vi "TimeResolvedSpectroscopy.vi"() -> ()   [LabVIEW 2016]
uses:
  C:/Users/VaidaLabAdmin/Desktop/CodyEthanJordan/LaserControl/DelayStageDlls/Thorlabs.MotionControl.Controls.dll
  DelayStageDlls/Thorlabs.MotionControl.Controls.dll
  C:/Users/VaidaLabAdmin/Desktop/CodyEthanJordan/LaserControl/DelayStageDlls/Thorlabs.MotionControl.Benchtop.BrushlessMotorCLI.dll
  DelayStageDlls/Thorlabs.MotionControl.Benchtop.BrushlessMotorCLI.dll
  C:/Users/VaidaLabAdmin/Desktop/CodyEthanJordan/LaserControl/DelayStageDlls/Thorlabs.MotionControl.GenericMotorCLI.dll
  DelayStageDlls/Thorlabs.MotionControl.GenericMotorCLI.dll
panel:
  out "Start Time":string="120419_1643"
  out "RoiSum":dbl=1907.0
  in  "Main UI":T1(tab)=enum."Collect Data"
  in  "BenchtopBrushlessControl 3":refnum<k24>(container)
  in  "SerialNumber":string="73871558"
  out "Settings":T2={"Range"=5056, "cftfak"=39321856, "RoiMin"=0, "RoiMax"=4096, "#Regions"=0, "Caluse"=1, "Calpoints"=0, "Param"=0, "Offset"=0, "Xdim"=0, "bitshift"=0, "Active"=1, "Roipreset"=0.0, "dummy1"=0.0, "dummy2"=0.0, "dummy3"=0.0} {"dummy3" format="%.2f"; "dummy2" format="%.2f"; "bitshift" format="%.0x"; "Active" format="%.0x"; "Offset" format="%.0x"; "Param" format="%.0x"; "dummy1" format="%.2f"; "Roipreset" format="%.2f"; "cftfak" format="%.0x"}
  in  "Maximum Scan\nPosition":dbl=3000.0
  out "Harmonics":cluster{"Y":dbl[], "Y":dbl[]}[](graph)=[{"Y"=[20.0], "Y"=[1907.0]}]
  in  "Start Scan":bool
  out "Spectrum":u32[](graph)
  in  "State":T3(ring)=enum."Move Grating"
  out "Delay Position":dbl=20.0
  in  "Step Size":dbl=10.0
  in  "Sweeps":i32=3000
  out "CHN Status":T4={"Started"=3, "Maxval"=0, "Runtime"=0.101, "Fifo full"=0.0, "TotalSum"=2383.0, "RoiSum"=1907.0, "Roirate"=5639.14373088685, "Sweeps"=3005.0, "Starts"=0.0, "Dummy"=0.0} {"Dummy" format="%.2f"; "Starts" format="%.2f"; "Sweeps" format="%.2f"; "Roirate" format="%.2f"; "RoiSum" format="%.2f"; "TotalSum" format="%.2f"; "Fifo full" format="%.2f"; "Runtime" format="%.2f"}
  in  "Photoelectron Spectra Destination":path=path "C:/Users/VaidaLabAdmin/Documents/TOF-PES/04-12-2019/test"
  out "Halt Confirmation":string="OK"
  out "MCSADat Error":i32
  in  "Spectrum #":i32
  in  "Stop":bool
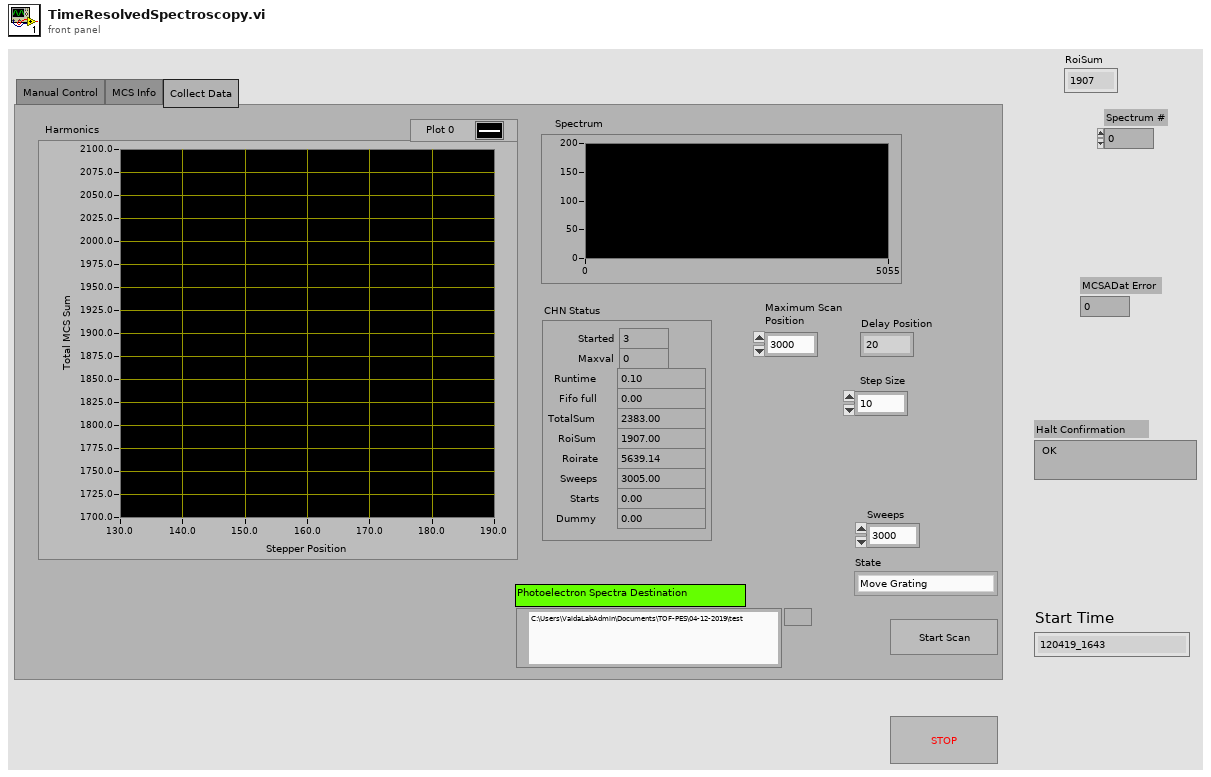
[diagram p1: front panel]
types:
  T1 = enum32{"Manual Control", "MCS Info", "Collect Data"}
  T2 = cluster{"Range":i32, "cftfak":i32, "RoiMin":i32, "RoiMax":i32, "#Regions":i32, "Caluse":i32, "Calpoints":i32, "Param":i32, "Offset":i32, "Xdim":i32, "bitshift":i32, "Active":i32, "Roipreset":dbl, "dummy1":dbl, "dummy2":dbl, "dummy3":dbl}
  T3 = enum16{"Start", "Move Grating", "Start MCS", "Collect Data", "Stop MCS", "Save Data", "Stop"}
  T4 = cluster{"Started":i32, "Maxval":u32, "Runtime":dbl, "Fifo full":dbl, "TotalSum":dbl, "RoiSum":dbl, "Roirate":dbl, "Sweeps":dbl, "Starts":dbl, "Dummy":dbl}
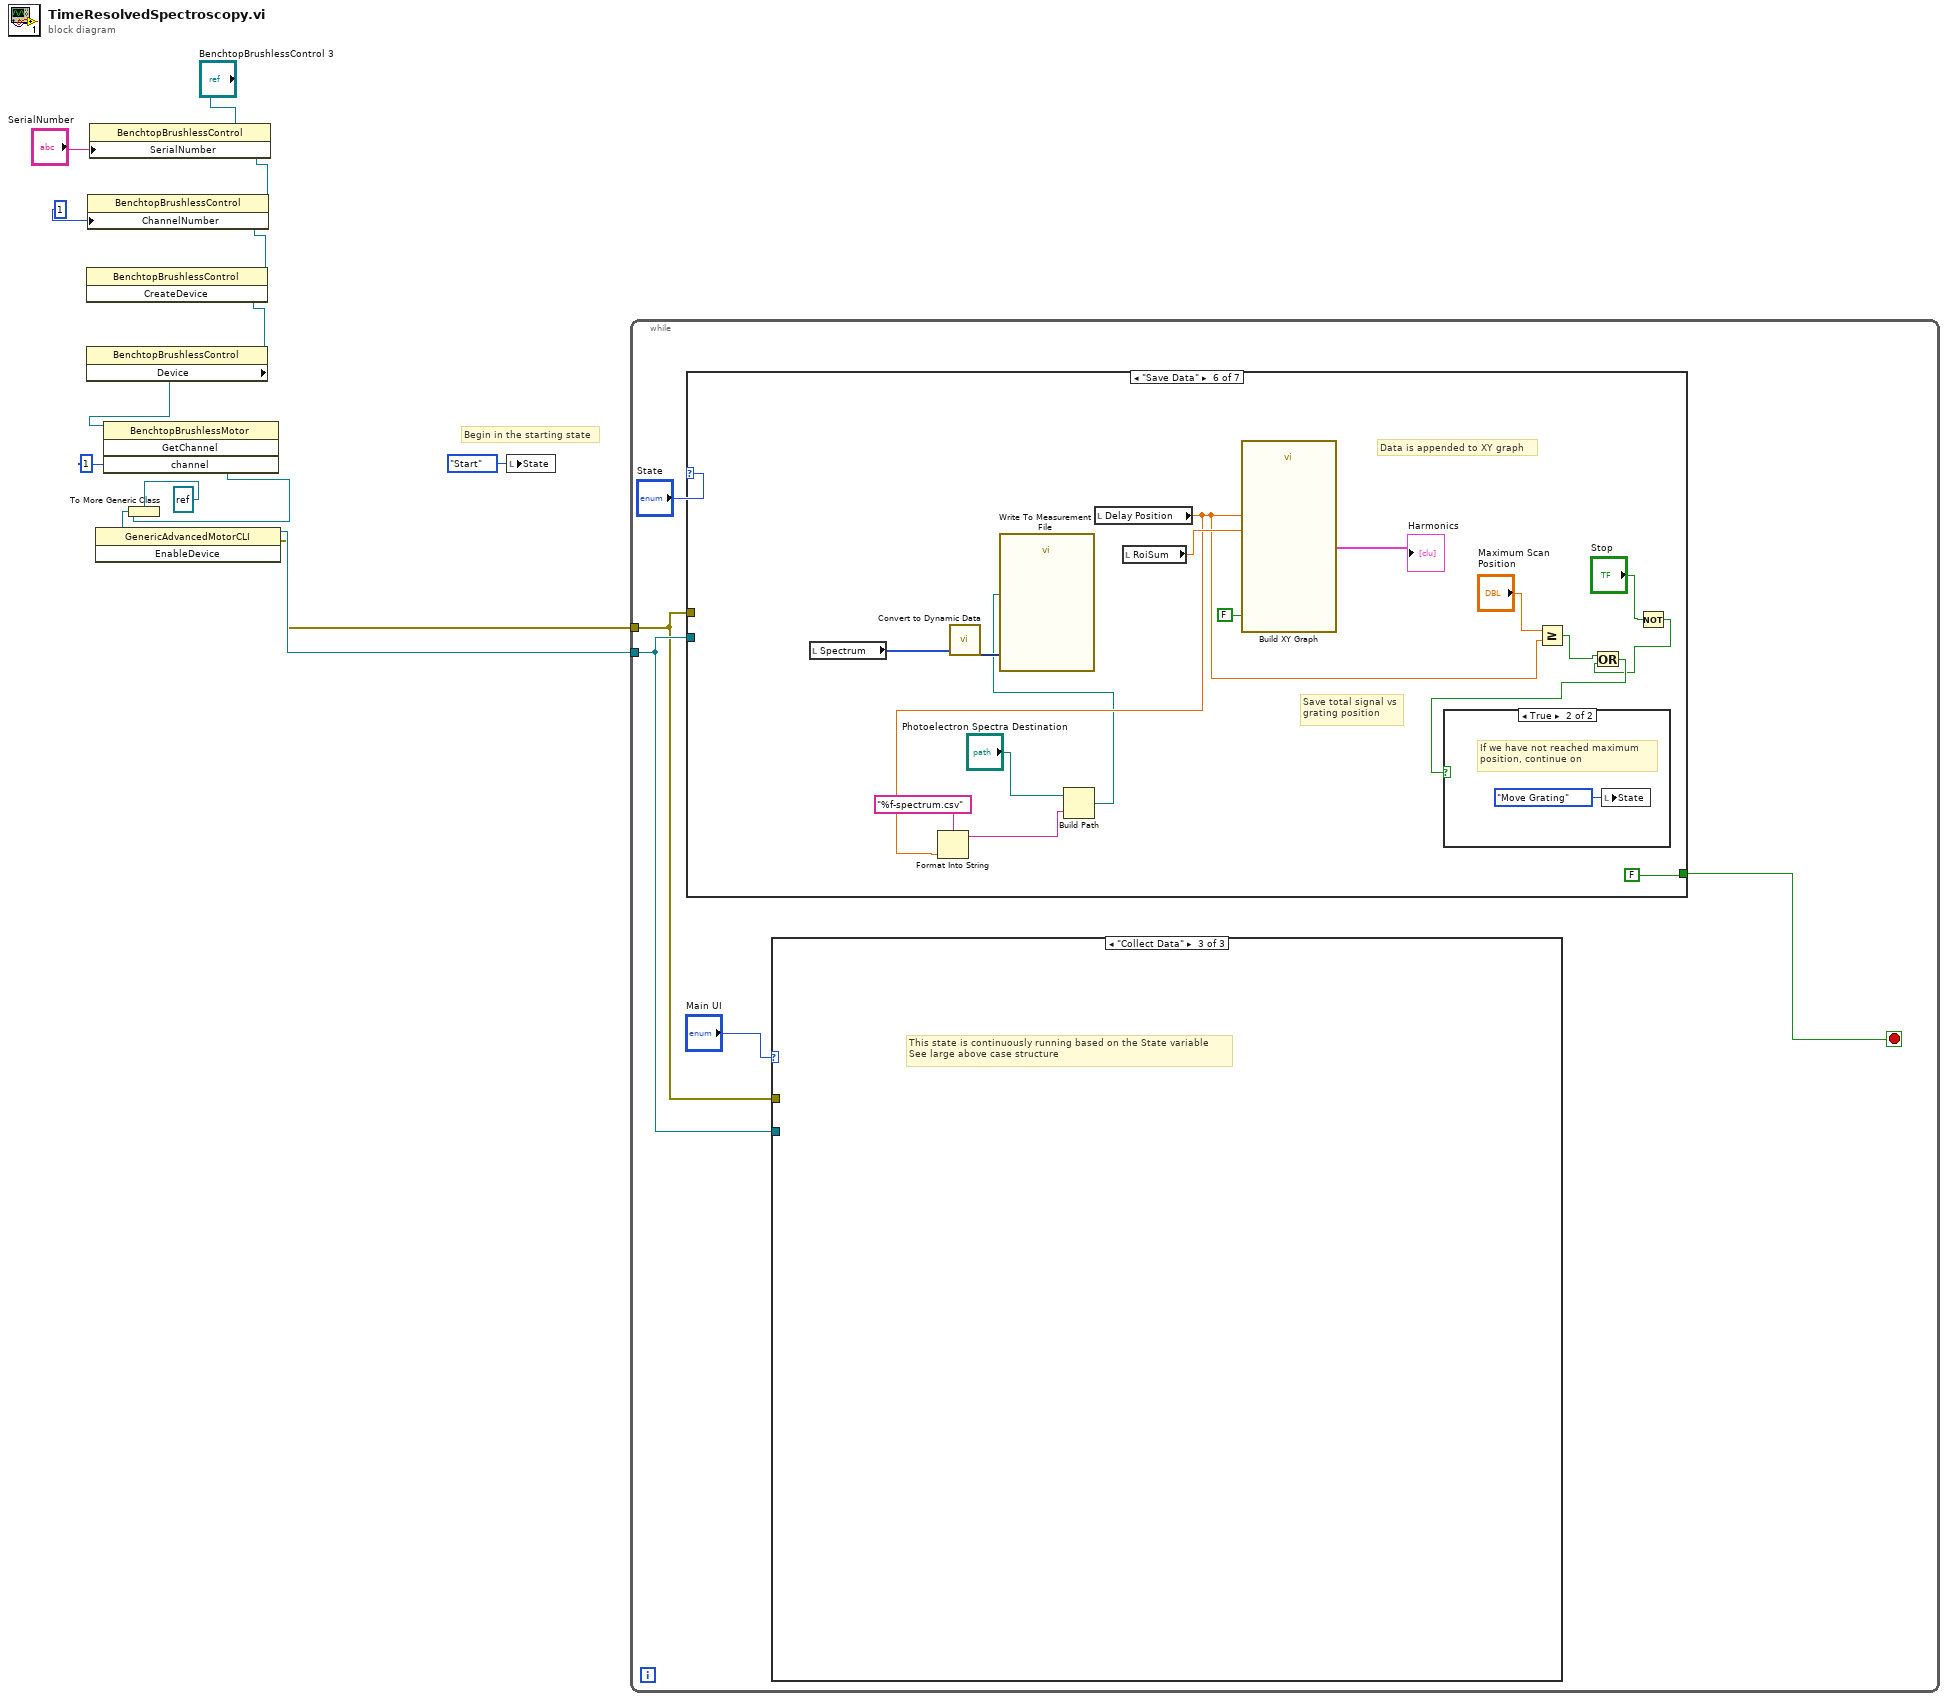
[diagram p0: block diagram]
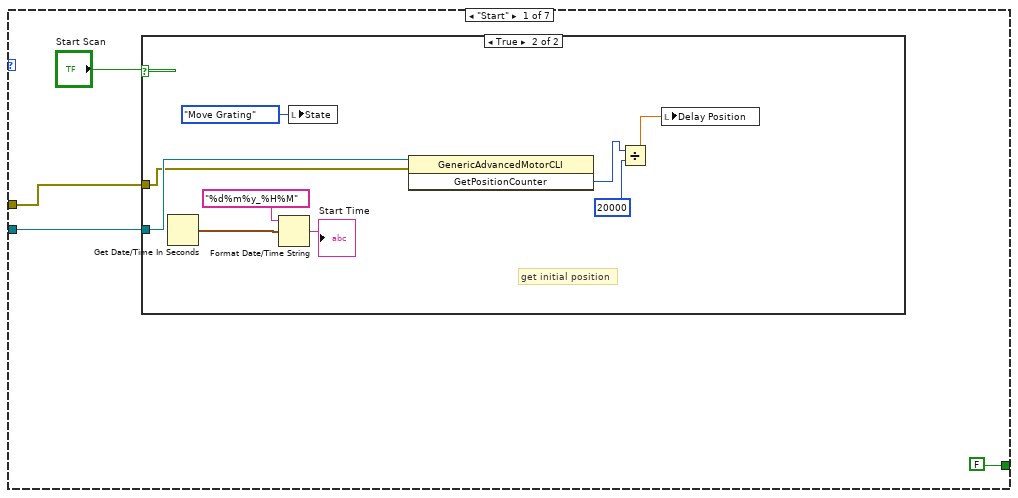
[diagram p4: hidden frame]
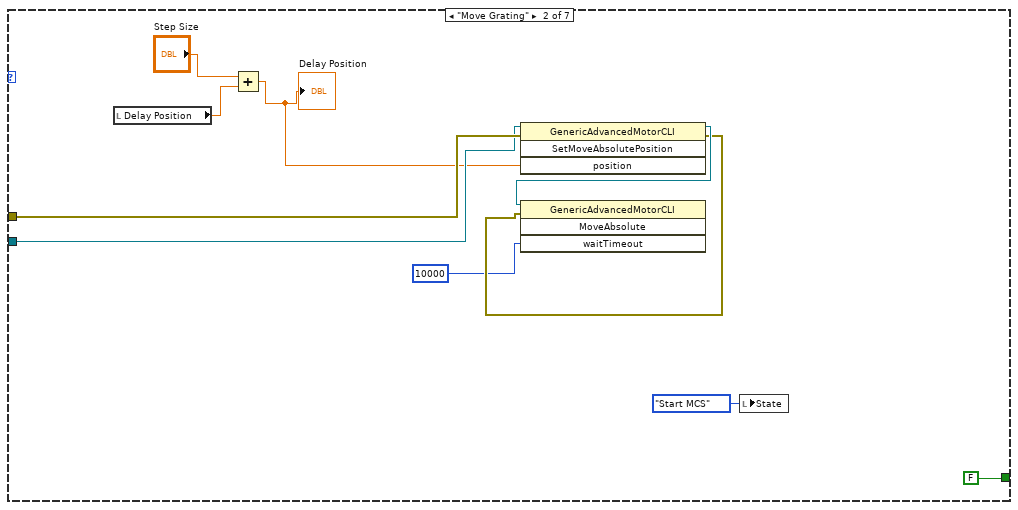
[diagram p6: hidden frame]
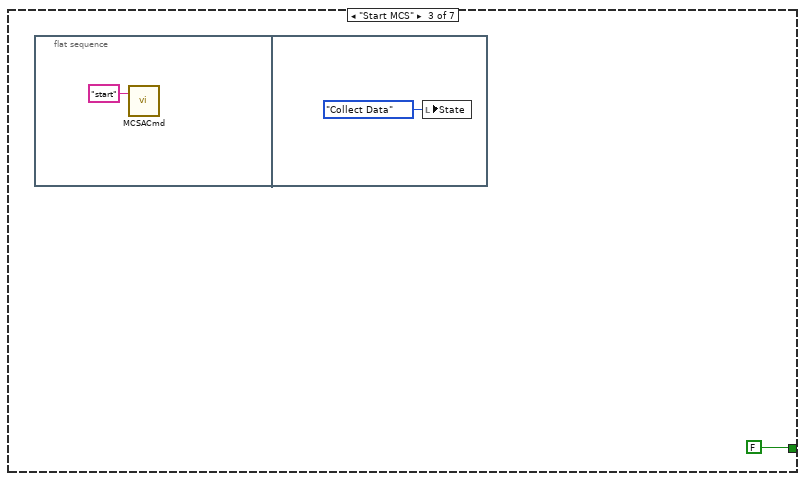
[diagram p7: hidden frame]
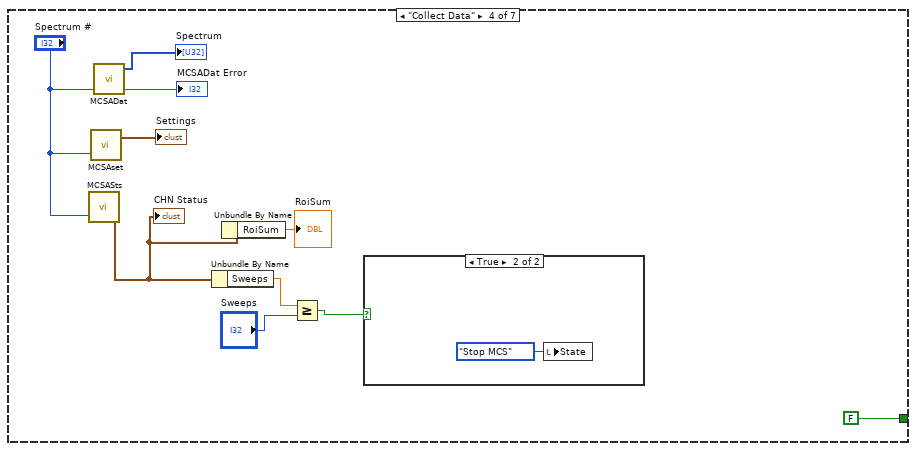
[diagram p8: hidden frame]
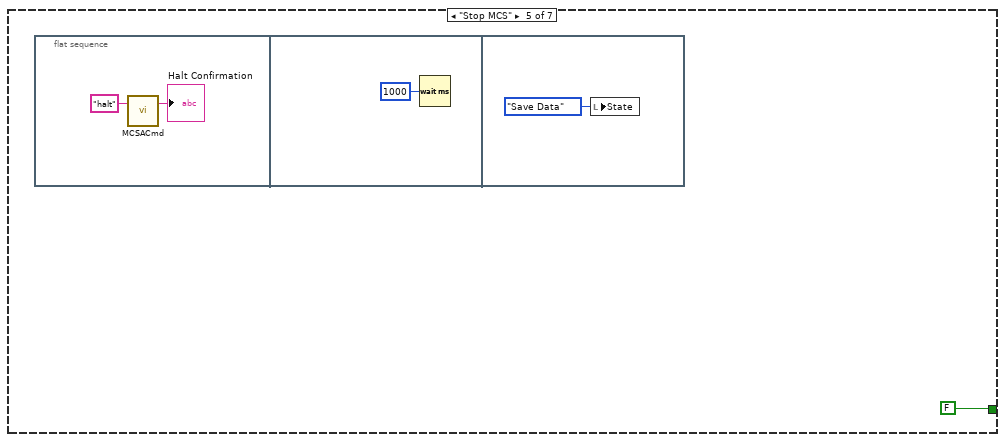
[diagram p10: hidden frame]
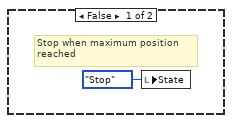
[diagram p11: hidden frame]
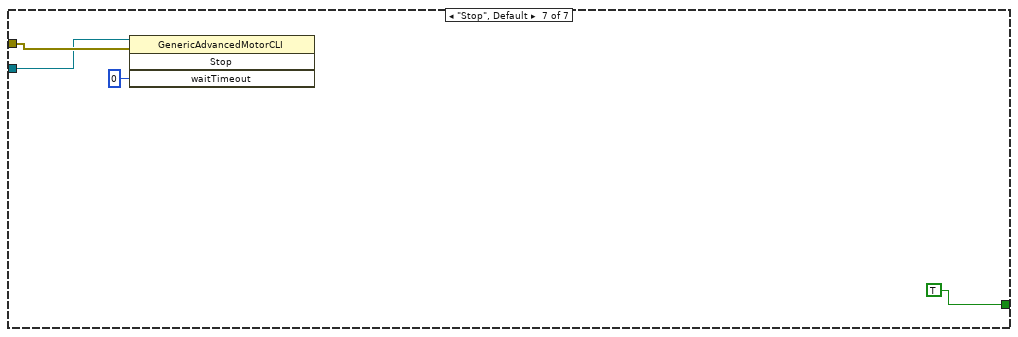
[diagram p12: hidden frame]
diagram:
  # "Begin in the starting state"
  n1 = property class="BenchtopBrushlessControl"(reference="BenchtopBrushlessControl 3", "SerialNumber"="SerialNumber") -> (reference out=w9:refnum<k24>)  [unwired: 1 in, 1 out]
  n2 = property class="BenchtopBrushlessControl"(reference=w9, "ChannelNumber"=1) -> (reference out=w8:refnum<k24>)  [unwired: 1 in, 1 out]
  n3 = invoke class="BenchtopBrushlessControl" method="CreateDevice"(reference=w8) -> (reference out=w7:refnum<k24>)  [unwired: 2 in, 2 out]
  n4 = property class="BenchtopBrushlessControl"(reference=w7) -> ("Device"=w6:refnum<k24>)  [unwired: 1 in, 2 out]
  n5 = invoke class="BenchtopBrushlessMotor" method="GetChannel"(reference=w6, "channel"=i16 1) -> ("GetChannel"=w4:refnum<k24>)  [unwired: 2 in, 3 out]
  n6 = To More Generic Class(target class=refnum<k24> refnum, reference=w4) -> (generic class reference=w5:refnum<k24>)
  n7 = invoke class="GenericAdvancedMotorCLI" method="EnableDevice"(reference=w5) -> (reference out=w2:refnum<k24>, error out=w1:errorcluster)  [unwired: 2 in, 1 out]
  n8 = local write "State"(T3."Start" ("State")) -> ()
  n9 = while {
    tunnel: w1 -> [w16]
    tunnel: w2 -> [w17]
    stop <- w15 stop-if-true
    n10 = case shown="\"Save Data\"" "State" {
      tunnel: w16 -> [w21 w38 _ _ _ _ w82]
      tunnel: w17 -> [w20 w36 _ _ _ _ w81]
      tunnel: [FALSE FALSE FALSE FALSE FALSE FALSE TRUE] -> w15
      frame "Start" {
        n11 = case shown="True" "Start Scan" {
          tunnel: w21 -> [_ w27]
          tunnel: w20 -> [_ w28]
          frame False {
          }
          frame True {
            # "get initial position"
            n12 = Get Date/Time In Seconds() -> (seconds since 1Jan1904=w30:timestamp)
            n13 = Format Date/Time String(time format string (%c)="%d%m%y_%H%M", seconds (now)=w30) -> (date/time string=→"Start Time":string)  [unwired: 1 in]
            n14 = local write "State"(T3."Move Grating" ("State")) -> ()
            n15 = invoke class="GenericAdvancedMotorCLI" method="GetPositionCounter"(reference=w28, error in=w27) -> ("GetPositionCounter"=w25:i32)  [unwired: 1 in, 2 out]
            n16 = Divide(x=w25, y=20000) -> (x/y=w26:dbl)
            n17 = local write "Delay Position"(w26) -> ()
          }
        }
      }
      frame "Move Grating" {
        n18 = local read "Delay Position"() -> (w41:dbl)
        n19 = Add(x="Step Size", y=w41) -> (x+y=w33:dbl)
        "Delay Position" <- w33
        n20 = invoke class="GenericAdvancedMotorCLI" method="SetMoveAbsolutePosition"(reference=w36, error in=w38, "position"=w33) -> (reference out=w39:refnum<k24>, error out=w37:errorcluster)  [unwired: 1 in, 2 out]
        n21 = invoke class="GenericAdvancedMotorCLI" method="MoveAbsolute"(reference=w39, error in=w37, "waitTimeout"=10000) -> ()  [unwired: 1 in, 4 out]
        n22 = local write "State"(T3."Start MCS" ("State")) -> ()
      }
      frame "Start MCS" {
        n23 = flat-sequence {
          frame #0 {
            n24 = call "MCSACmd.vi"("Command"="start") -> ()  [unwired: 2 in, 1 out]
          }
          frame #1 {
            n25 = local write "State"(T3."Collect Data" ("State")) -> ()
          }
        }
      }
      frame "Collect Data" {
        n26 = call "MCSASts.vi"("CHN #"="Spectrum #") -> ("CHN Status"=w48:T4)  [unwired: 1 in, 1 out]
        "CHN Status" <- w48
        n27 = call "MCSAset.vi"("Spect #"="Spectrum #") -> ("Settings"=→"Settings":T2)  [unwired: 1 in, 1 out]
        n28 = call "MCSADat.vi"("Spectrum #"="Spectrum #") -> ("MCSADat Error"=→"MCSADat Error":i32, "Data"=→"Spectrum":u32[])  [unwired: 2 in, 1 out]
        n29 = Unbundle By Name(w48) -> ("Sweeps"=w51:dbl)
        n30 = Unbundle By Name(w48) -> ("RoiSum"=→"RoiSum":dbl)
        n31 = Greater Or Equal?(x=w51, y="Sweeps") -> (x >= y?=w49:bool)
        n32 = case shown="True" w49 {
          frame False {
            # "Do nothing, continue\ncollecting data"
          }
          frame True {
            n33 = local write "State"(T3."Stop MCS" ("State")) -> ()
          }
        }
      }
      frame "Stop MCS" {
        n34 = flat-sequence {
          frame #0 {
            n35 = call "MCSACmd.vi"("Command"="halt") -> ("Response"=→"Halt Confirmation":string)  [unwired: 2 in]
          }
          frame #1 {
            n36 = Wait (ms)(milliseconds to wait=u32 1000) -> ()  [unwired: 1 out]
          }
          frame #2 {
            n37 = local write "State"(T3."Save Data" ("State")) -> ()
          }
        }
      }
      frame "Save Data" {
        # "Data is appended to XY graph"
        # "Save total signal vs\ngrating position"
        n38 = local read "Spectrum"() -> (w64:u32[])
        n39 = call "Convert to Dynamic Data"("Array"=w64) -> ("Dynamic Data Type"=w63:dynamicdata)  [unwired: 3 in]
        n40 = local read "Delay Position"() -> (w67:dbl)
        n41 = Format Into String(format string="%f-spectrum.csv", w67) -> (resulting string=w65:string)  [unwired: 2 in, 1 out]
        n42 = Build Path(base path="Photoelectron Spectra Destination", name or relative path=w65) -> (appended path=w62:path)
        n43 = call "Write To Measurement File"("Signals"=w63, "Filename"=w62) -> ()  [unwired: 15 in, 3 out]
        n44 = local read "RoiSum"() -> (w75:dbl)
        n45 = call "Build XY Graph"("Reset"=FALSE, "Y Input"=w75, "X Input"=w67) -> ("XY Graph"=→"Harmonics":cluster{"X":dbl[], "Y":dbl[]}[])  [unwired: 7 in, 1 out]
        n46 = Greater Or Equal?(x="Maximum Scan\nPosition", y=w67) -> (x >= y?=w71:bool)
        n47 = Not(x="Stop") -> (.not. x?=w68:bool)
        n48 = Or(x=w71, y=w68) -> (x .or. y?=w70:bool)
        n49 = case shown="True" w70 {
          frame False {
            # "Stop when maximum position\nreached"
            n50 = local write "State"(T3."Stop" ("State")) -> ()
          }
          frame True {
            # "If we have not reached maximum\nposition, continue on"
            n51 = local write "State"(T3."Move Grating" ("State")) -> ()
          }
        }
      }
      frame "Stop", Default {
        n52 = invoke class="GenericAdvancedMotorCLI" method="Stop"(reference=w81, error in=w82, "waitTimeout"=0) -> ()  [unwired: 1 in, 4 out]
      }
    }
    n53 = case shown="\"Collect Data\"" "Main UI" {
      tunnel: w17 -> [_ _ _]
      tunnel: w16 -> [_ _ _]
      frame "Manual Control", Default {
      }
      frame "MCS Info" {
        # "Ensure MCS6A.exe is running and that the 32/64 bit version of LabView matches the version of the MCS\nsoftware running, most setup done through that program\n\nIn particular set a Sweeps Preset under Hardware Options to be the desired sweeps + 1"
      }
      frame "Collect Data" {
        # "This state is continuously running based on the State variable\nSee large above case structure"
      }
    }
  }
